vi "Start RAD.vi"() -> ()   [LabVIEW 2020]
panel:
  out "error out":errorcluster
  # "Opening The Replication And Deployment Utility..."
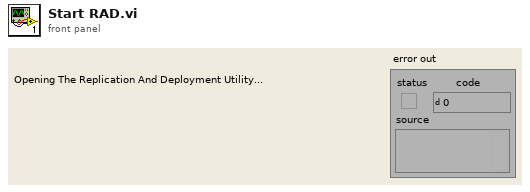
[diagram p1: front panel]
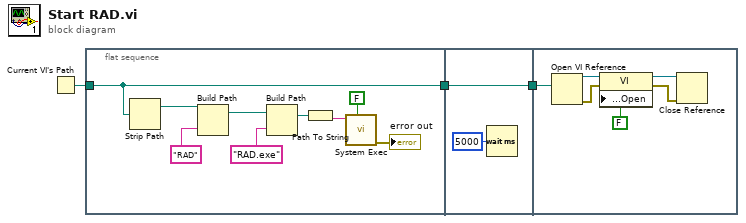
[diagram p0: block diagram]
diagram:
  n1 = Current VI's Path() -> (path=w1:path)
  n2 = flat-sequence {
    tunnel: [w4] -> w2
    tunnel: w1 -> [w4]
    tunnel: [w14] -> w3
    tunnel: w2 -> [w14]
    tunnel: w3 -> [w17]
    frame #0 {
      n3 = Strip Path(path=w4) -> (stripped path=w11:path)  [unwired: 1 out]
      n4 = Build Path(base path=w11, name or relative path="RAD") -> (appended path=w9:path)
      n5 = Build Path(base path=w9, name or relative path="RAD.exe") -> (appended path=w7:path)
      n6 = Path To String(path=w7) -> (string=w12:string)
      n7 = call <vilib>:"System Exec.vi"("wait until completion? (T)"=FALSE, "command line"=w12) -> ("error out"=→"error out":errorcluster)  [unwired: 6 in, 3 out]
    }
    frame #1 {
      n8 = Wait (ms)(milliseconds to wait=u32 5000) -> ()  [unwired: 1 out]
    }
    frame #2 {
      n9 = Open VI Reference(vi path=w17) -> (vi reference=w19:refnum<vi>, error out=w20:errorcluster)  [unwired: 5 in]
      n10 = property class="VI"(reference=w19, error in=w20, "Front Panel.Open"=FALSE) -> (reference out=w16:refnum<vi>, error out=w15:errorcluster)
      n11 = Close Reference(reference=w16, error in (no error)=w15) -> ()  [unwired: 1 out]
    }
  }
